vi "tango_labview.vi"(9 "previous":T1, 10 "i":i64, 11 "archive":T1) -> (0 "error out":errorcluster)   [LabVIEW 2020]
uses:
  archive.ctl
  sync_type_def.ctl
  HT_type-def.ctl
  HF_type_def.ctl
  vacuum_type_def.ctl
  modulator_type_def.ctl
  water_cooling_type_def.ctl
  all_magnets_type_def.ctl
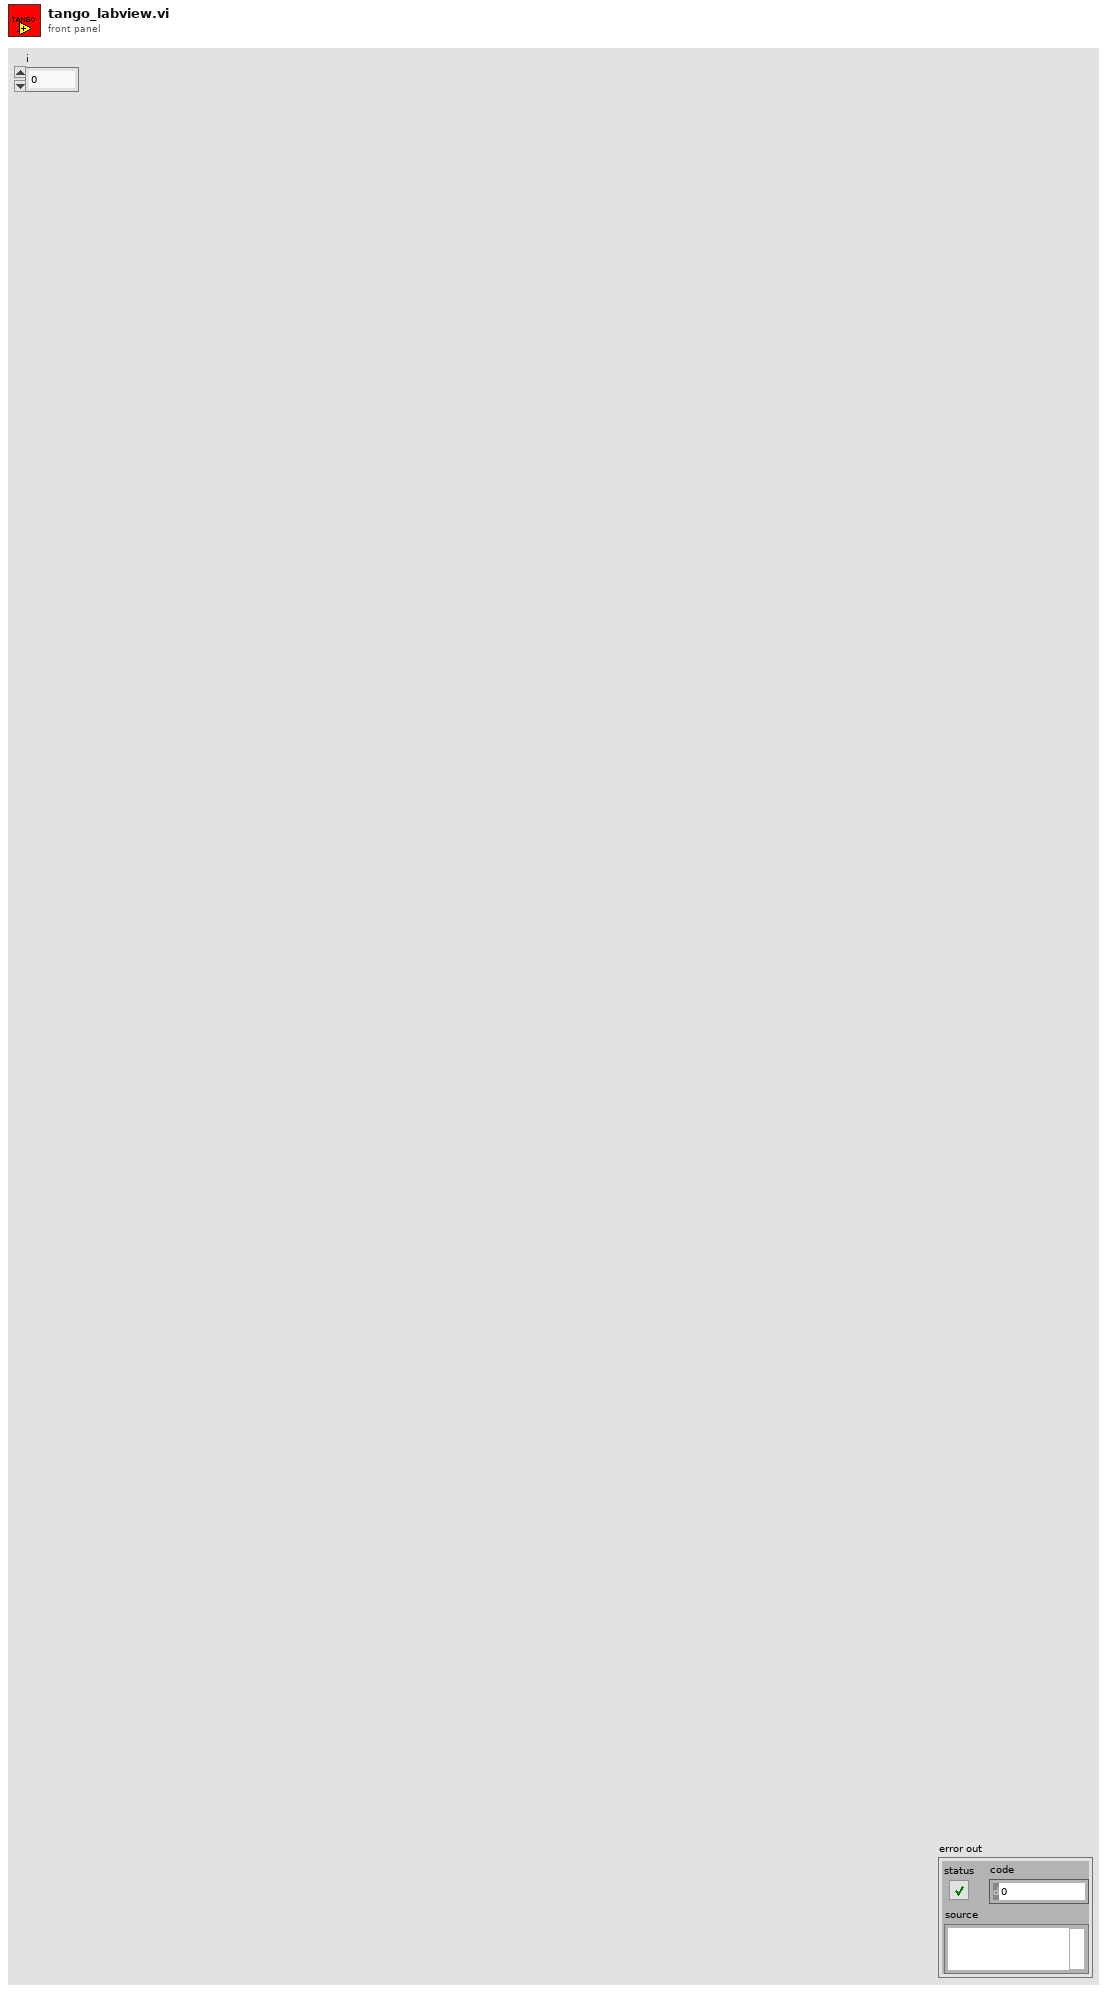
[diagram p1: front panel]
types:
  T1 = typedef "archive.ctl" = cluster{"sync":T2, "HT":T3, "HF":T4, "vacuum":T5, "modulator":T6, "cooling":T7, "magnets":T8, "time":cluster{"elyse/timestamp":dbl}}
  T2 = typedef "sync_type_def.ctl" = cluster{"elyse/sync/NI6071E/delay":dbl, "elyse/sync/NI6071E/width":dbl, "elyse/sync/frequency/delay":dbl, "elyse/sync/frequency/width":dbl, "elyse/sync/WCM/delay":dbl, "elyse/sync/WCM/width":dbl, "elyse/sync/modulator/delay":dbl, "elyse/sync/modulator/width":dbl, "elyse/sync/HF/delay":dbl, "elyse/sync/HF/width":dbl, "elyse/sync/Faraday/delay":dbl, "elyse/sync/Faraday/width":dbl, "elyse/sync/Oscilloscope/delay":dbl, "elyse/sync/Oscilloscope/width":dbl, "elyse/sync/50Hz_20MHz/delay":dbl, "elyse/sync/50Hz_20MHz/width":dbl, "elyse/sync/laser_HF/delay":dbl, "elyse/sync/laser_HF/width":dbl, "elyse/sync/IMAC/delay":dbl, "elyse/sync/IMAC/width":dbl, "elyse/sync/laser/delay":dbl, "elyse/sync/laser/width":dbl, "elyse/sync/oscilloscope1/delay":dbl, "elyse/sync/oscilloscope1/width":dbl, "elyse/sync/oscilloscope2/delay":dbl, "elyse/sync/oscilloscope2/width":dbl, "elyse/sync/detection1/delay":dbl, "elyse/sync/detection1/width":dbl, "elyse/sync/detection1/delay":dbl, "elyse/sync/detection2/width":dbl, "elyse/sync/machine/delay":dbl, "elyse/sync/machine/width":dbl, "elyse/sync/n_selection":dbl}
  T3 = typedef "HT_type-def.ctl" = cluster{"elyse/HT/voltage/set_value":dbl, "elyse/HT/voltage/value":dbl, "elyse/HT/current/value":dbl, "elyse/preamplifier/set_value":dbl, "elyse/preamplifier/value":dbl}
  T4 = typedef "HF_type_def.ctl" = cluster{"elyse/HF/attenuator/value":dbl, "elyse/HF/dephaser/value":dbl, "elyse/HF/dephaser/value_manuel":dbl, "elyse/HF/canon/value":dbl, "elyse/HF/section/value":dbl}
  T5 = typedef "vacuum_type_def.ctl" = cluster{"elyse/vacuum/preparation_chamber/state":bool, "elyse/vacuum/preparation_chamber/measurement":dbl, "elyse/vacuum/HF/state":bool, "elyse/vacuum/HF/measurement":dbl, "elyse/vacuum/canon/state":bool, "elyse/vacuum/canon/measurement":dbl, "elyse/vacuum/section/state":bool, "elyse/vacuum/section/measurement":dbl, "elyse/vacuum/dipole1/state":bool, "elyse/vacuum/dipole1/measurement":dbl, "elyse/vacuum/screen1/state":bool, "elyse/vacuum/screen1/measurement":dbl, "elyse/vacuum/mirror/state":bool, "elyse/vacuum/mirror/measurement":dbl, "elyse/vacuum/tpg300_section/state":bool, "elyse/vacuum/tpg300_section/measurement":dbl, "elyse/vacuum/valves/cathode/state":bool, "elyse/vacuum/valves/injection/state":bool}
  T6 = typedef "modulator_type_def.ctl" = cluster{"elyse/modulator/focale1/current/value":dbl, "elyse/modulator/focale2/current/value":dbl, "elyse/modulator/focale3/current/value":dbl, "elyse/modulator/LAR/voltage/value":dbl, "elyse/modulator/line_end/current/value":dbl, "elyse/modulator/thyratron/currents/power/value":dbl, "elyse/modulator/thyratron_reservoir/current/value":dbl, "elyse/modulator/paramagnetization/current/value":dbl, "elyse/modulator/thyratron/voltages/heating/value":dbl, "elyse/modulator/thyratron/currents/heating/value":dbl, "elyse/modulator/klystron/currents/power/value":dbl, "elyse/modulator/klystron/voltages/power/value":dbl, "elyse/modulator/klystron/currents/heating/value":dbl, "elyse/modulator/klystron/voltages/heating/value":dbl}
  T7 = typedef "water_cooling_type_def.ctl" = cluster{"elyse/cooling/section/temperature/set_value":dbl, "elyse/cooling/section/temperature/measurement":dbl, "elyse/cooling/canon/temperature/set_value":dbl, "elyse/cooling/canon/temperature/measurement":dbl}
  T8 = typedef "all_magnets_type_def.ctl" = cluster{"elyse/magnets/focale/set_value":dbl, "elyse/magnets/focale/value":dbl, "elyse/magnets/phase_HF_laser/set_value":dbl, "elyse/magnets/phase_HF_laser/value":dbl, "elyse/magnets/dipole1/set_value":dbl, "elyse/magnets/dipole1/value":dbl, "elyse/magnets/dipole2/set_value":dbl, "elyse/magnets/dipole2/value":dbl, "elyse/magnets/Cor_H1/set_value":dbl, "elyse/magnets/Cor_H1/value":dbl, "elyse/magnets/Cor_V1/set_value":dbl, "elyse/magnets/Cor_V1/value":dbl, "elyse/magnets/Cor_H2/set_value":dbl, "elyse/magnets/Cor_H2/value":dbl, "elyse/magnets/Cor_V2/set_value":dbl, "elyse/magnets/Cor_V2/value":dbl, "elyse/magnets/Cor_H3/set_value":dbl, "elyse/magnets/Cor_H3/value":dbl, "elyse/magnets/Cor_V3/set_value":dbl, "elyse/magnets/Cor_V3/value":dbl, "elyse/magnets/Cor_H4/set_value":dbl, "elyse/magnets/Cor_H4/value":dbl, "elyse/magnets/Cor_V4/set_value":dbl, "elyse/magnets/Cor_V4/value":dbl, "elyse/magnets/Cor_H5/set_value":dbl, "elyse/magnets/Cor_H5/value":dbl, "elyse/magnets/Cor_V5/set_value":dbl, "elyse/magnets/Cor_V5/value":dbl, "elyse/magnets/triplet1-1/set_value":dbl, "elyse/magnets/triplet1-1/value":dbl, "elyse/magnets/triplet1-2/set_value":dbl, "elyse/magnets/triplet1-2/value":dbl, "elyse/magnets/triplet2-1/set_value":dbl, "elyse/magnets/triplet2-1/value":dbl, "elyse/magnets/triplet2-2/set_value":dbl, "elyse/magnets/triplet2-2/value":dbl, "elyse/magnets/qudrupole1/set_value":dbl, "elyse/magnets/qudrupole1/value":dbl, "elyse/magnets/qudrupole2/set_value":dbl, "elyse/magnets/qudrupole2/value":dbl}
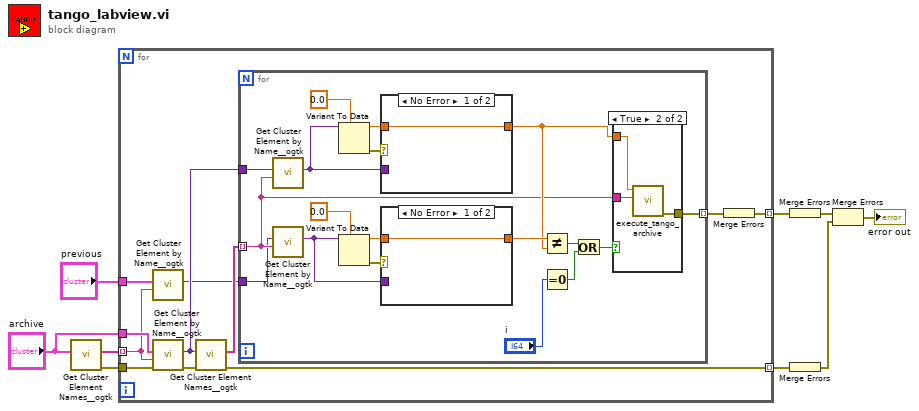
[diagram p0: block diagram]
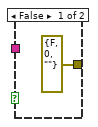
[diagram p2: hidden frame]
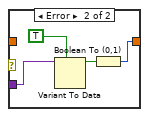
[diagram p3: hidden frame]
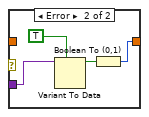
[diagram p4: hidden frame]
diagram:
  n1 = call <userlib>:"Get Cluster Element Names__ogtk.vi"("Cluster"="archive") -> ("error out"=w9:errorcluster, "Element Names"=w7:string[])  [unwired: 9 in]
  n2 = for {
    tunnel: w7 -> [w13] mode=indexing
    tunnel: "archive" -> [w20]
    tunnel: w9 -> [w18]
    tunnel: [w17] -> w5 mode=indexing
    tunnel: "previous" -> [w14]
    tunnel: [w10] -> w4 mode=indexing
    n3 = call <userlib>:"Get Cluster Element by Name__ogtk.vi"("Element Name"=w13, "Cluster"=w14) -> ("VElement"=w12:variant)  [unwired: 7 in, 2 out]
    n4 = call <userlib>:"Get Cluster Element by Name__ogtk.vi"("error in (no error)"=w18, "Element Name"=w13, "Cluster"=w20) -> ("error out"=w19:errorcluster, "VElement"=w15:variant)  [unwired: 6 in, 1 out]
    n5 = call <userlib>:"Get Cluster Element Names__ogtk.vi"("error in (no error)"=w19, "Cluster"=w15) -> ("error out"=w17:errorcluster, "Element Names"=w16:string[])  [unwired: 8 in]
    n6 = for {
      tunnel: w16 -> [w23] mode=indexing
      tunnel: w15 -> [w37]
      tunnel: w12 -> [w22]
      tunnel: [w24] -> w11 mode=indexing
      n7 = call <userlib>:"Get Cluster Element by Name__ogtk.vi"("Element Name"=w23, "Cluster"=w37) -> ("VElement"=w35:variant)  [unwired: 7 in, 2 out]
      n8 = call <userlib>:"Get Cluster Element by Name__ogtk.vi"("Element Name"=w23, "Cluster"=w22) -> ("VElement"=w21:variant)  [unwired: 7 in, 2 out]
      n9 = Variant To Data(type=0.0, Variant=w35) -> (data=w34:dbl, error out=w36:errorcluster)  [unwired: 1 in]
      n10 = Variant To Data(type=0.0, Variant=w21) -> (data=w33:dbl, error out=w32:errorcluster)  [unwired: 1 in]
      n11 = case shown="No Error" w36 {
        tunnel: w35 -> [_ w52]
        tunnel: [w48 w49] -> w27
        tunnel: w34 -> [w48 _]
        frame No Error {
        }
        frame Error {
          n12 = Variant To Data(type=TRUE, Variant=w52) -> (data=w50:bool)  [unwired: 1 in, 1 out]
          n13 = Boolean To (0,1)(Boolean=w50) -> (0, 1=w49:i16)
        }
      }
      n14 = case shown="No Error" w32 {
        tunnel: w21 -> [_ w47]
        tunnel: [w43 w44] -> w28
        tunnel: w33 -> [w43 _]
        frame No Error {
        }
        frame Error {
          n15 = Variant To Data(type=TRUE, Variant=w47) -> (data=w45:bool)  [unwired: 1 in, 1 out]
          n16 = Boolean To (0,1)(Boolean=w45) -> (0, 1=w44:i16)
        }
      }
      n17 = Not Equal?(x=w28, y=w27) -> (x != y?=w26:bool)
      n18 = Equal To 0?(x="i") -> (x = 0?=w29:bool)
      n19 = Or(x=w26, y=w29) -> (x .or. y?=w25:bool)
      n20 = case shown="True" w25 {
        tunnel: w23 -> [_ w42]
        tunnel: w27 -> [_ w41]
        tunnel: [errorcluster {"status"=FALSE, "code"=0, "source"=""} ("error out") w40] -> w24
        frame False {
        }
        frame True {
          n21 = call "execute_tango_archive.vi"("Data Name"=w42, "Numeric"=w41) -> ("error out"=w40:errorcluster)  [unwired: 9 in]
        }
      }
    }
    n22 = Merge Errors(w11) -> (w10:errorcluster)
  }
  n23 = Merge Errors(w4) -> (w3:errorcluster)
  n24 = Merge Errors(w5) -> (w2:errorcluster)
  n25 = Merge Errors(w3, w2) -> (→"error out":errorcluster)
